vi "Save Data.vi"(8 "灵敏度":dbl, 9 "测量数据":string[][](table), 10 "历史数据":string[][](table), 11 "AI信号":dbl(graph)) -> (0 "数据输出":string[][](array[string]), 1 "要保存的数据":string[][](array[string]), 3 "文件名":string)   [LabVIEW 2016]
panel:
  out "数组":string[][](array[string])
  out "Row":i32
  in  "取消":bool
  in  "确定":bool
  out "项符号":i32[](array[numeric])
  out "选择要保存的数据":i32(listbox)
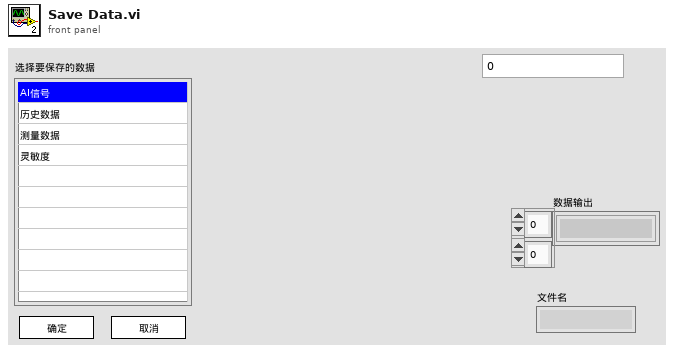
[diagram p1: front panel]
types:
  T1 = typedef "LVPoint32TypeDef.ctl" = cluster{"Horizontal":i32, "Vertical":i32}
  T2 = typedef "LVRowAndColumnTypeDef.ctl" = cluster{"Row":i32, "Column":i32}
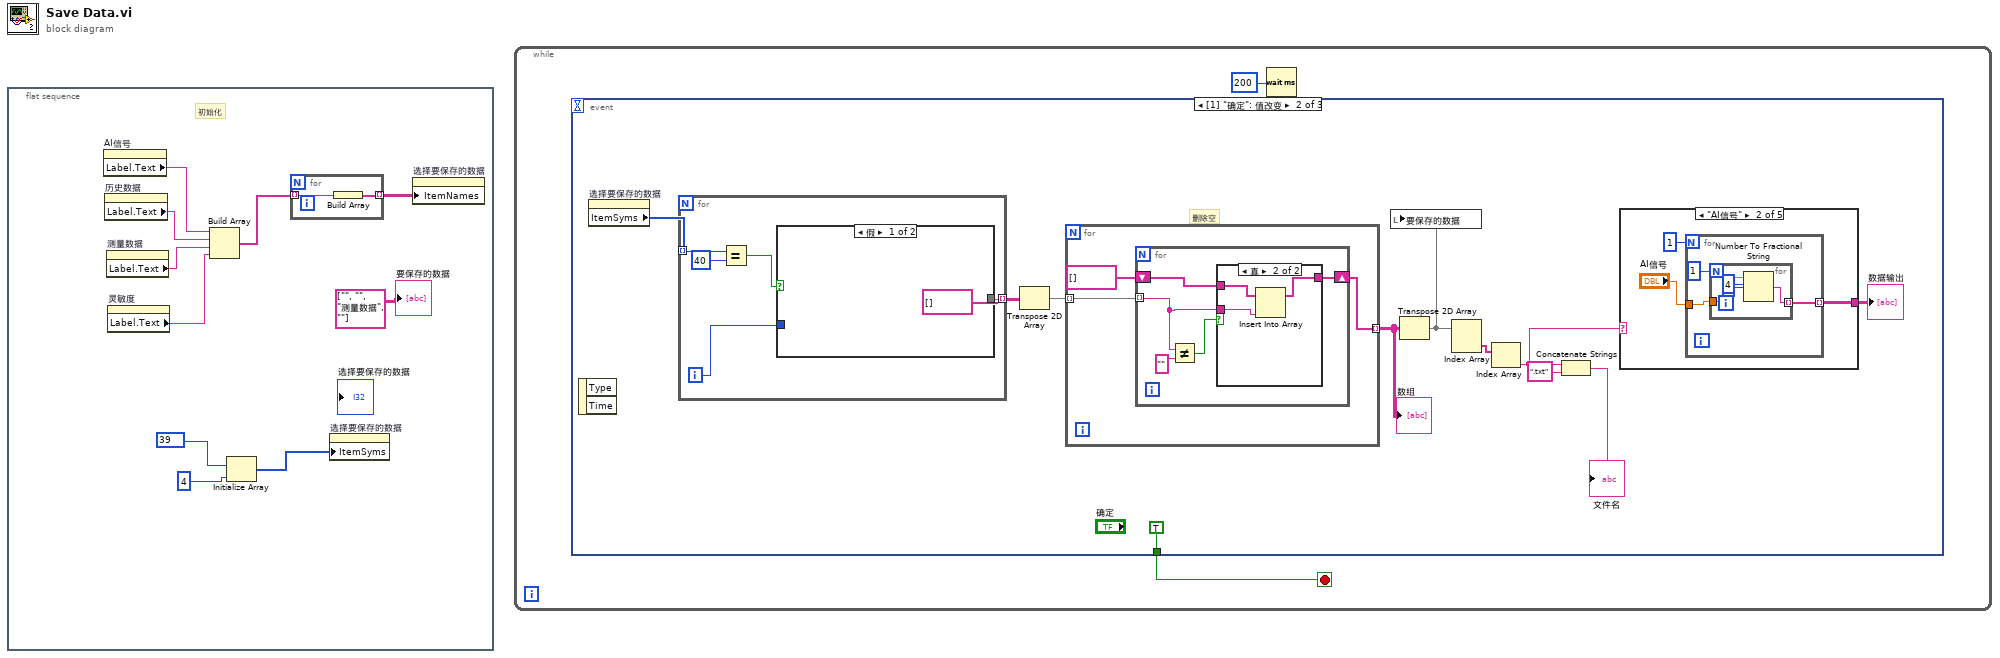
[diagram p0: block diagram]
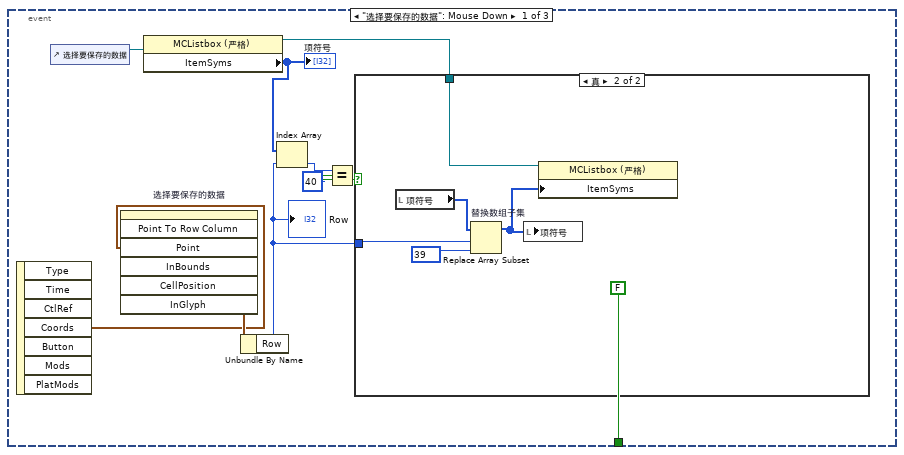
[diagram p2: hidden frame]
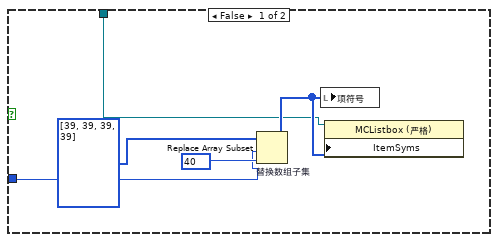
[diagram p3: hidden frame]
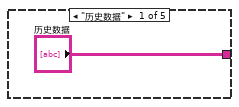
[diagram p4: hidden frame]
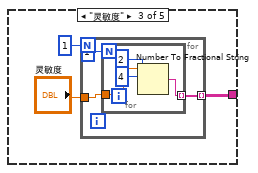
[diagram p5: hidden frame]
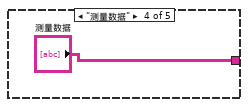
[diagram p6: hidden frame]
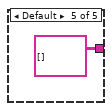
[diagram p7: hidden frame]
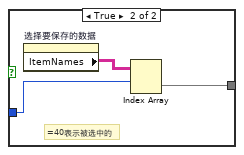
[diagram p9: hidden frame]
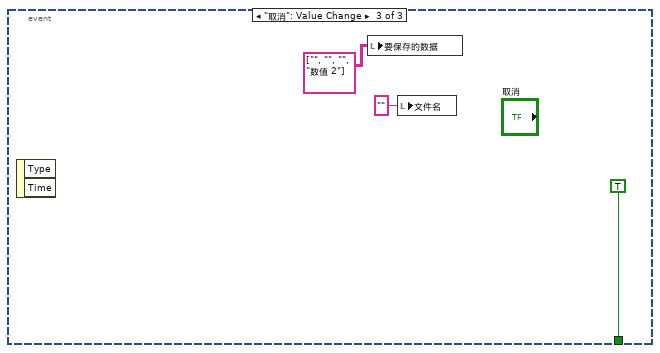
[diagram p10: hidden frame]
diagram:
  n1 = flat-sequence {
    frame #0 {
      # "初始化"
      n2 = property on="AI信号" class="WFChart (strict)"() -> ("Label.Text"=w10:string)  [unwired: 2 in, 2 out]
      n3 = property on="历史数据" class="Tbl (strict)"() -> ("Label.Text"=w9:string)  [unwired: 2 in, 2 out]
      n4 = property on="测量数据" class="Tbl (strict)"() -> ("Label.Text"=w8:string)  [unwired: 2 in, 2 out]
      n5 = property on="灵敏度" class="DigNum (strict)"() -> ("Label.Text"=w7:string)  [unwired: 2 in, 2 out]
      n6 = Build Array(w10, w9, w8, w7) -> (w6:string[])
      n7 = Initialize Array(39, 4) -> (w2:i32[])
      n8 = for {
        tunnel: w6 -> [w12] mode=indexing
        tunnel: [w11] -> w5 mode=indexing
        n9 = Build Array(w12) -> (w11:string[])
      }
      n10 = property on="选择要保存的数据" class="MCListbox (strict)"("ItemSyms"=w2) -> ()  [unwired: 2 in, 2 out]
      n11 = property on="选择要保存的数据" class="MCListbox (strict)"("ItemNames"=w5) -> ()  [unwired: 2 in, 2 out]
      "要保存的数据" <- string[][] [[""], [""], ["测量数据"], [""]] ("要保存的数据")
    }
  }
  n12 = while {
    stop <- w14 stop-if-true
    n13 = event shown="[1] \"确定\": 值改变" {
      selector: _ -> [_ _ _]
      dyn-events: _ -> [_ _ _]
      timeout: _ -> [_ _ _]
      tunnel: [FALSE TRUE TRUE] -> w14
      event "选择要保存的数据": Mouse Down {
        n14 = event-data() -> ("Coords"=w17:T1)  [unwired: 1 in, 6 out]
        n15 = control-ref of="选择要保存的数据"() -> (w23:refnum<vi>)
        n16 = invoke on="选择要保存的数据" class="MCListbox (严格)" method="Point To Row Column"("Point"=w17) -> ("CellPosition"=w18:T2)  [unwired: 6 in, 6 out]
        n17 = property class="MCListbox (严格)"(reference=w23) -> (reference out=w22:refnum<vi>, "ItemSyms"=w15:i32[])  [unwired: 1 in, 1 out]
        "项符号" <- w15
        n18 = Unbundle By Name(w18) -> ("Row"=w16:i32)
        "Row" <- w16
        n19 = Index Array(array=w15, index=w16) -> (element=w19:i32)
        n20 = Equal?(x=w19, y=40) -> (x = y?=w21:bool)
        n21 = case shown="真" w21 {
          tunnel: w22 -> [w27 w31]
          tunnel: w16 -> [w26 w30]
          frame False {
            n22 = Replace Array Subset "替换数组子集"(array=i32[] [39, 39, 39, 39], new element=40, index=w26) -> (w28:i32[])
            n23 = local write "项符号"(w28) -> ()
            n24 = property class="MCListbox (严格)"(reference=w27, "ItemSyms"=w28) -> ()  [unwired: 1 in, 2 out]
          }
          frame True {
            n25 = local read "项符号"() -> (w34:i32[])
            n26 = Replace Array Subset "替换数组子集"(array=w34, new element=39, index=w30) -> (w32:i32[])
            n27 = local write "项符号"(w32) -> ()
            n28 = property class="MCListbox (严格)"(reference=w31, "ItemSyms"=w32) -> ()  [unwired: 1 in, 2 out]
          }
        }
      }
      event "确定": Value Change {
        # "删除空"
        n29 = event-data() -> ()  [unwired: 1 in, 2 out]
        n30 = property on="选择要保存的数据" class="MCListbox (strict)"() -> ("ItemSyms"=w44:i32[])  [unwired: 2 in, 2 out]
        n31 = for {
          tunnel: w44 -> [w85] mode=indexing
          tunnel: [w81] -> w42 mode=indexing
          i -> [w82]
          n32 = Equal?(x=w85, y=40) -> (x = y?=w83:bool)
          n33 = case shown="假" w83 {
            tunnel: w82 -> [_ w88]
            tunnel: [string[] [] ("ItemNames") w87] -> w81
            frame False {
            }
            frame True {
              # "=40表示被选中的"
              n34 = property on="选择要保存的数据" class="MCListbox (strict)"() -> ("ItemNames"=w89:string[][])  [unwired: 2 in, 2 out]
              n35 = Index Array(array=w89, index (row)=w88) -> (element=w87:string[])  [unwired: 1 in]
            }
          }
        }
        n36 = Transpose 2D Array(2D array=w42) -> (transposed array=w41:string[][])
        n37 = for {
          tunnel: w41 -> [w71] mode=indexing
          tunnel: [w69] -> w43 mode=indexing
          n38 = for {
            tunnel: w71 -> [w73] mode=indexing
            shift-right: [w72] -> w69
            shift-left: string[] [] -> [w74]
            n39 = Not Equal?(x=w73, y="") -> (x != y?=w75:bool)
            n40 = case shown="真" w75 {
              tunnel: w74 -> [w77 w80]
              tunnel: w73 -> [_ w79]
              tunnel: [w77 w78] -> w72
              frame False {
              }
              frame True {
                n41 = Insert Into Array(array=w80, new element=w79) -> (w78:string[])  [unwired: 1 in]
              }
            }
          }
        }
        "数组" <- w43
        n42 = Transpose 2D Array(2D array=w43) -> (transposed array=w37:string[][])
        n43 = local write "要保存的数据"(w37) -> ()
        n44 = Index Array(array=w37) -> (element=w40:string[])  [unwired: 2 in]
        n45 = Index Array(array=w40) -> (element=w38:string)  [unwired: 1 in]
        n46 = Concatenate Strings(w38, ".txt" ("字符串")) -> (→"文件名":string)
        n47 = case shown="\"AI信号\"" w38 {
          tunnel: ["历史数据" w48 w58 "测量数据" string[][] [] ("测量数据")] -> w35
          frame "历史数据" {
          }
          frame "AI信号" {
            n48 = for {
              N: 1 -> [_]
              tunnel: "AI信号" -> [w52]
              tunnel: [w51] -> w48 mode=indexing
              n49 = for {
                N: 1 -> [_]
                tunnel: w52 -> [w56]
                tunnel: [w54] -> w51 mode=indexing
                n50 = Number To Fractional String(number=w56, width (-)=i16 2 ("宽度(-)"), precision (6)=i16 4 ("精度(6)")) -> (F-format string=w54:string)  [unwired: 1 in]
              }
            }
          }
          frame "灵敏度" {
            n51 = for {
              N: 1 -> [_]
              tunnel: "灵敏度" -> [w62]
              tunnel: [w61] -> w58 mode=indexing
              n52 = for {
                N: 1 -> [_]
                tunnel: w62 -> [w66]
                tunnel: [w64] -> w61 mode=indexing
                n53 = Number To Fractional String(number=w66, width (-)=i16 2 ("宽度(-)"), precision (6)=i16 4 ("精度(6)")) -> (F-format string=w64:string)  [unwired: 1 in]
              }
            }
          }
          frame "测量数据" {
          }
          frame Default {
          }
        }
        "数据输出" <- w35
      }
      event "取消": Value Change {
        n54 = event-data() -> ()  [unwired: 1 in, 2 out]
        n55 = local write "要保存的数据"(string[][] [[""], [""], [""], ["数值 2"]] ("要保存的数据")) -> ()
        n56 = local write "文件名"("" ("文件名")) -> ()
      }
    }
    n57 = Wait (ms)(milliseconds to wait=u32 200 ("等待时间（毫秒）")) -> ()  [unwired: 1 out]
  }
